vi "BNC555.set i Attr and create DIM Services.vi"(0 "i ref in":refnum<vi>, 5 "error in (no error)":errorcluster) -> (14 "i ref out":refnum<vi>, 17 "i Attributes":T1={"Information"={"VISA resource name"="", "Baud Rate (1:9600)"=1}, "Channel Array"=[], "System"={"Sys Period"=0.0, "Sys Oscillator"=FALSE, "Sys Mode"=enum."Normal", "Sys Burst #"=0, "Sys DC On"=10, "Sys DC Off"=5, "Sys Trig Mode"=enum."Gated", "Sys Trig Lev"=2.5, "Sys Gate State"=TRUE, "Sys Trig Edge"=TRUE, "Sys State"=TRUE}, "GUI Refs"={"Delete"=refnum, "Information"=refnum, "System"=refnum, "Channel Array"=refnum, "Device Error"=refnum, "Instr Driver Revision"=refnum, "Instr Firmware Revision"=refnum, "Instr Option"=refnum, "Self-Test Response"=refnum}, "Service IDs Channelinfo"=[-1], "Service ID T0 Mode"=-1} {"System"."Sys Period" format="%.6p"; "System"."Sys Trig Lev" format="%.4p"; "Channel Array"."Chan Lev Adjust" format="%.3p"; "Channel Array"."Chan Width" format="%.3p"; "Channel Array"."Chan Delay" format="%.3p"; "Channel Array"."Chan #" items=["System (To)", "Channel A", "Channel B", "Channel C", "Channel D", "Channel E", "Channel F", "Channel G", "Channel H"]; "Information"."Baud Rate (1:9600)" items=["4800", "9600", "19200", "38400"]}, 19 "error out":errorcluster)   [LabVIEW 2014, in "BNC555.lvlib"]
doc: "This VI gets database information to be stored in own attributes and starts a DIM service."
uses:
  BNC555.lvlib
  BNC555.i attribute.ctl
  non_GPL/instr.lib/BNC555/BNC555_U.llb/BNC555 All Chan Parameters.ctl
  non_GPL/instr.lib/BNC555/BNC555_U.llb/BNC555 All Sys Parameters.ctl
  CSPhelix/PH_Common/PH_Common.lvlib
  non_GPL/instr.lib/BNC555/BNC555 - Driver np.lvlib
  CSCore/CSSystem/CSSystemLib/CSSystemLib.lvlib
panel:
  # "Run\nStop"
  # "System (To) Mode"
  # "Triggering"
  # "High\nLow"
  # "Rising\nFalling"
  # "External\nInternal"
  # "Output"
  # "Gate"
  # "On\nOff"
  # "Pulse"
  # "On\nOff"
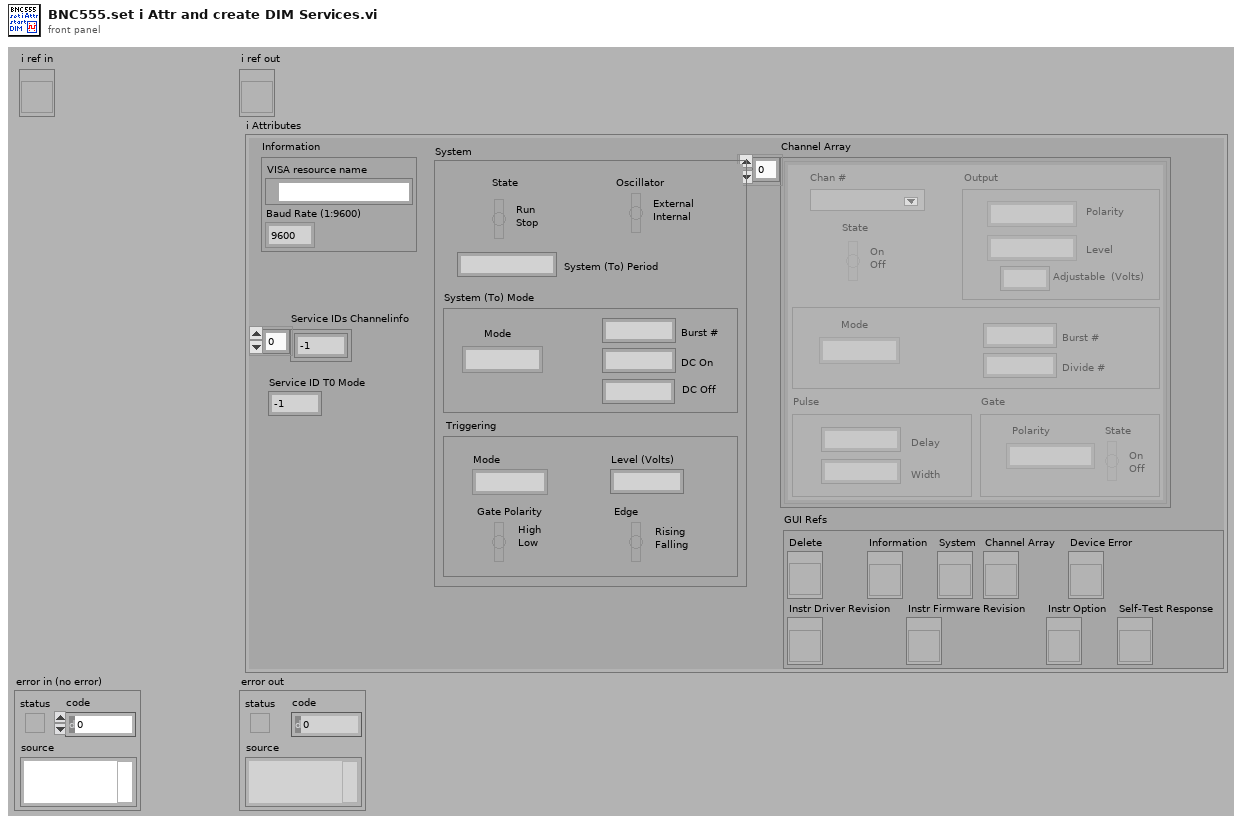
[diagram p1: front panel]
types:
  T1 = typedef "BNC555.lvlib/BNC555.i attribute.ctl" = cluster{"Information":cluster{"VISA resource name":refnum<visa-resource-name>, "Baud Rate (1:9600)":u16}, "Channel Array":T2[], "System":T3, "GUI Refs":cluster{"Delete":refnum<vi>, "Information":refnum<vi>, "System":refnum<vi>, "Channel Array":refnum<vi>, "Device Error":refnum<vi>, "Instr Driver Revision":refnum<vi>, "Instr Firmware Revision":refnum<vi>, "Instr Option":refnum<vi>, "Self-Test Response":refnum<vi>}, "Service IDs Channelinfo":i32[], "Service ID T0 Mode":i32}
  T2 = typedef "BNC555 - Driver np.lvlib/BNC555 All Chan Parameters.ctl" = cluster{"Chan #":i32, "Chan State":bool, "Chan Delay":dbl, "Chan Width":dbl, "Chan Mode":enum16{"Normal", "Single", "Burst", "Divide by N"}, "Chan Burst #":u32, "Chan Divide #":u32, "Chan Pol Out":enum16{"Normal", "Complement", "Inverted"}, "Chan Level Out":enum16{"TTL", "Adjustable", "35 Volt"}, "Chan Lev Adjust":dbl, "Chan Gate Pol":enum16{"Normal", "Complement", "Inverted"}, "Chan Gate State":bool}
  T3 = typedef "BNC555 - Driver np.lvlib/BNC555 All Sys Parameters.ctl" = cluster{"Sys Period":dbl, "Sys Oscillator":bool, "Sys Mode":enum16{"Normal", "Single", "Burst", "Duty Cycle"}, "Sys Burst #":u32, "Sys DC On":u32, "Sys DC Off":u32, "Sys Trig Mode":enum16{"Disabled", "Triggered", "Gated"}, "Sys Trig Lev":dbl, "Sys Gate State":bool, "Sys Trig Edge":bool, "Sys State":bool}
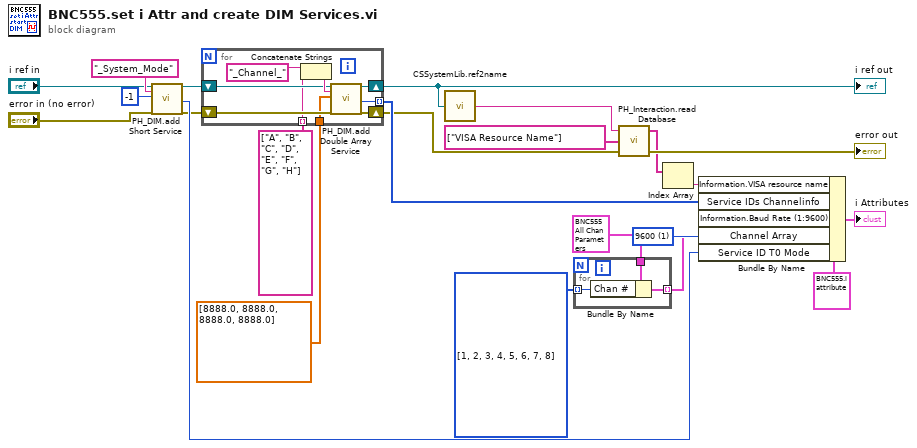
[diagram p0: block diagram]
diagram:
  w13 = i32[] [1, 2, 3, 4, 5, 6, 7, 8] items=["System (To)", "Channel A", "Channel B", "Channel C", "Channel D", "Channel E", "Channel F", "Channel G", "Channel H"]
  w15 = u16 1 items=["4800", "9600", "19200", "38400"] ("Baud Rate (1:9600)")
  n1 = call "PH_DIM.add Short Service.vi"("i ref in"="i ref in", "Service Name"="_System_Mode", "Number"=i16 -1, "error in (no error)"="error in (no error)") -> ("i ref out"=w2:refnum<vi>, "Service ID"=w16:i32, "error out"=w3:errorcluster)  [unwired: 13 in]
  n2 = for {
    shift-right: [w32] -> w4
    shift-left: w2 -> [w28]
    shift-right: [w30] -> w5
    shift-left: w3 -> [w31]
    tunnel: string[] ["A", "B", "C", "D", "E", "F", "G", "H"] -> [w26] mode=indexing
    tunnel: [w25] -> w22 mode=indexing
    tunnel: dbl[] [8888.0, 8888.0, 8888.0, 8888.0] ("Double Value Array") -> [w24]
    n3 = Concatenate Strings("_Channel_" ("string"), w26) -> (w29:string)
    n4 = call "PH_DIM.add Double Array Service.vi"("i ref in"=w28, "Service Name"=w29, "Double Value Array"=w24, "error in (no error)"=w31) -> ("i ref out"=w32:refnum<vi>, "Service ID"=w25:i32, "error out"=w30:errorcluster)  [unwired: 13 in]
  }
  "i ref out" <- w4
  n5 = call "CSSystemLib.ref2name.vi"("obj refnum"=w4) -> ("name"=w9:string)
  n6 = for {
    tunnel: T2 {"Chan #"=1, "Chan State"=TRUE, "Chan Delay"=0.01, "Chan Width"=0.01, "Chan Mode"=enum."Normal", "Chan Burst #"=10, "Chan Divide #"=10, "Chan Pol Out"=enum."Normal", "Chan Level Out"=enum."TTL", "Chan Lev Adjust"=5.0, "Chan Gate Pol"=enum."Normal", "Chan Gate State"=FALSE} ("Channel Parameters") -> [w35]
    tunnel: w13 -> [w34] mode=indexing
    tunnel: [w33] -> w12 mode=indexing
    n7 = Bundle By Name(cluster=w35, "Chan #"=w34) -> (w33:T2)
  }
  n8 = call "PH_Interaction.read Database.vi"("error in (no error)"=w5, "Strings to search for"=string[] ["VISA Resource Name"], "DB Entry to read"=w9) -> ("error out"=→"error out":errorcluster, "Values"=w8:string[])  [unwired: 1 in]
  n9 = Index Array(array=w8) -> (element=w7:string)  [unwired: 1 in]
  n10 = Bundle By Name(cluster=T1 {"Information"={"VISA resource name"="", "Baud Rate (1:9600)"=0}, "Channel Array"=[], "System"={"Sys Period"=0.0, "Sys Oscillator"=FALSE, "Sys Mode"=enum."Normal", "Sys Burst #"=0, "Sys DC On"=0, "Sys DC Off"=0, "Sys Trig Mode"=enum."Disabled", "Sys Trig Lev"=0.0, "Sys Gate State"=FALSE, "Sys Trig Edge"=FALSE, "Sys State"=FALSE}, "GUI Refs"={"Delete"=refnum, "Information"=refnum, "System"=refnum, "Channel Array"=refnum, "Device Error"=refnum, "Instr Driver Revision"=refnum, "Instr Firmware Revision"=refnum, "Instr Option"=refnum, "Self-Test Response"=refnum}, "Service IDs Channelinfo"=[], "Service ID T0 Mode"=0} ("i Attributes"), "Information.VISA resource name"=w7, "Service IDs Channelinfo"=w22, "Information.Baud Rate (1:9600)"=w15, "Channel Array"=w12, "Service ID T0 Mode"=w16) -> (→"i Attributes":T1)
